vi "test_output_freq_fpga.vi"() -> ()   [LabVIEW 2013]
uses:
  <vilib>/Platform/TimedLoop/XDataNode/timing_clust.ctl
  <vilib>/Platform/TimedLoop/XDataNode/nitl_modes.ctl
  <vilib>/Platform/TimedLoop/XDataNode/wakeup.ctl
  <vilib>/rvi/Emulation/niFpgaSctlEmulationGetInTimedLoop.vi
  <vilib>/rvi/Emulation/niFpgaEmulationReportErrorSimple.vi
  <vilib>/rvi/Emulation/niFpgaGetClockAttributes.vi
  <vilib>/rvi/eio/common/nirviEmuTemplateMethod_errors.vi
  <vilib>/rvi/Emulation/niFpgaCriticalErrorInLSC.vi
  <vilib>/Platform/TimedLoop/XDataNode/XDataNode.xnode
  <vilib>/eio/EIONode/EIONode.xnode
  <vilib>/rvi/FXPMathLib/FxpSub/XNode/nifxpmath_Sub.xnode
  <vilib>/Platform/TimedLoop/XDataNode/XDNodeRunTimeDep.lvlib
  <vilib>/rvi/FXPMathLib/sim/FxpSim.dll
panel:
  in  "samples per period":fxp<+,32,32>=1000000000.0
  in  "set samples":bool
  in  "User Command Commit":bool
  in  "User Command":u8
  out "User Command Idle":bool
  out "User Command Status":u8
  in  "User Data 0":u8
  in  "User Data 1":u8
  out "PLL Locked":bool
  out "User Error":bool
  out "Configured?":bool
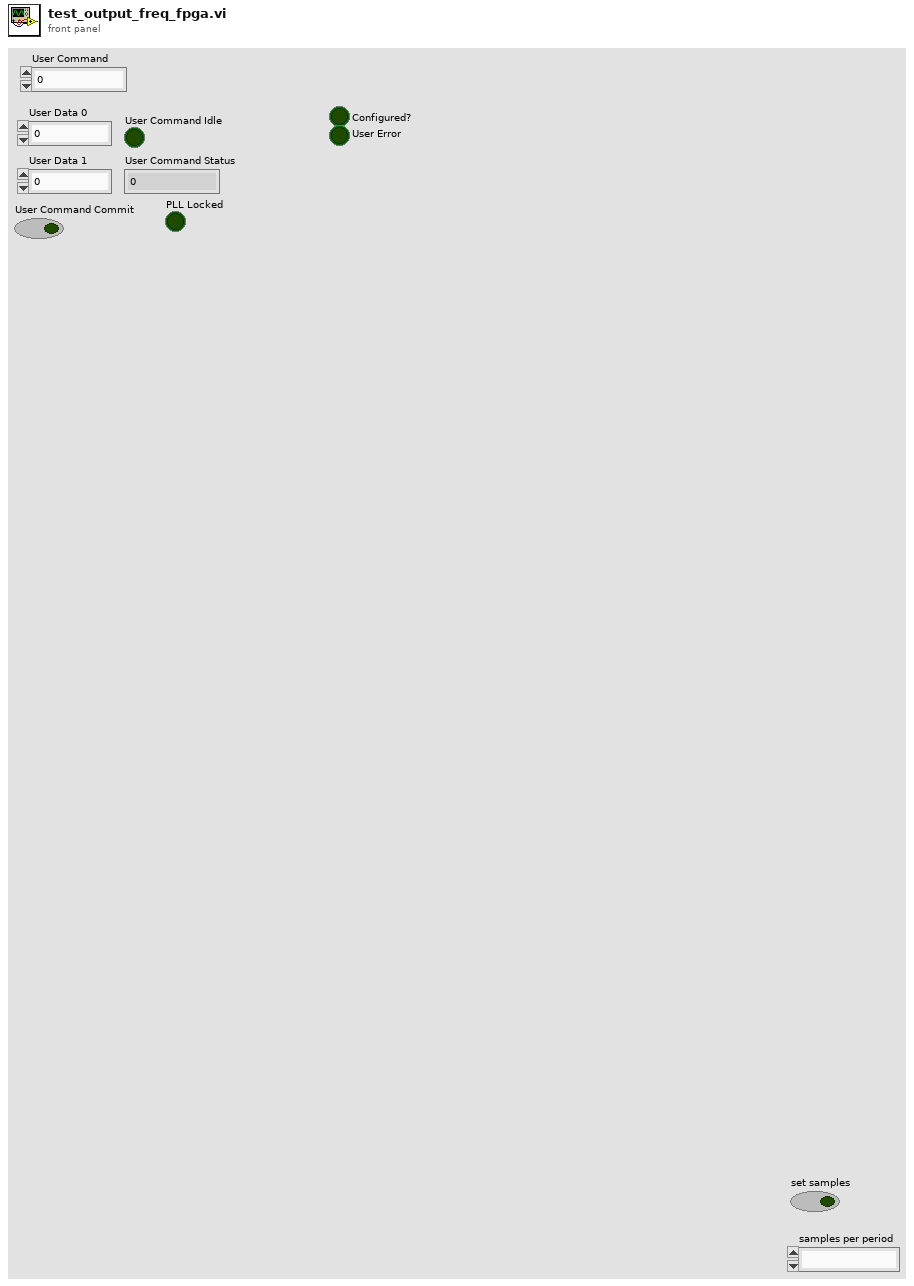
[diagram p1: front panel]
types:
  T1 = typedef "XDNodeRunTimeDep.lvlib/timing_clust.ctl" = cluster{"Expected End [f-1]":u64, "Actual End [f-1]":u64, "Finished Late? [f-1]":bool, "Expected End [i-1]":u64, "Actual End [i-1]":u64, "Finished Late? [i-1]":bool, "Expected Start [i]":u64, "Actual Start [i]":u64, "Expected Start [f]":u64, "Actual Start [f]":u64, "Source Name":string, "Structure Name":string, "Period":i64, "Deadline":i64, "Offset":i64, "Start":i64, "Priority":i32, "Timeout":i32, "Mode":T2, "Wakeup Reason":T3, "Error":errorcluster, "Source Type":string, "Secondary Source Type":string, "Global End Time":u64, "Global Start Time":u64, "Frame Duration":u64, "Iteration Duration":u64, "Assigned CPU":i32, "I/O Scan Engine Mode":u32}
  T2 = typedef "XDNodeRunTimeDep.lvlib/nitl_modes.ctl" = enum32{"No Change", "Process missed periods, maintain original phase", "Discard missed periods, maintain original phase", "Process missed periods, ignore original phase", "Discard missed periods, ignore original phase"}
  T3 = typedef "XDNodeRunTimeDep.lvlib/wakeup.ctl" = enum32{"Normal", "Aborted", "Asynchronous wakeup", "Timing source error", "Timed loop error", "Timeout"}
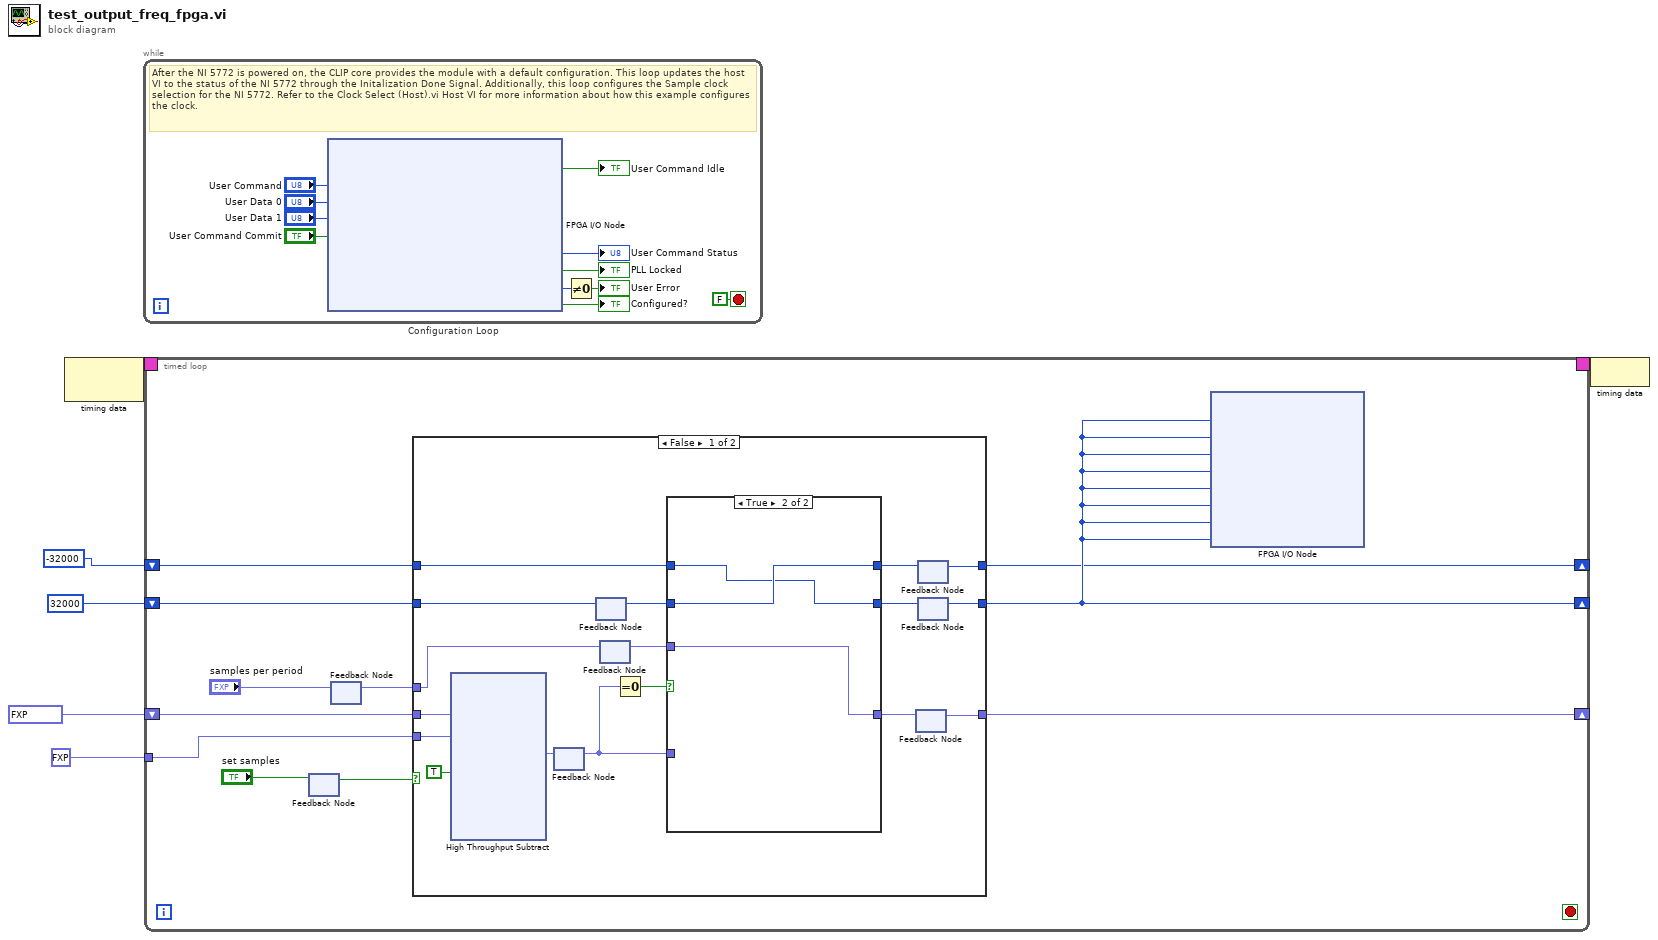
[diagram p0: block diagram]
diagram:
  n1 = node-c288() -> (w6:T1)  [unwired: 1 in]
  n2 = while "Configuration Loop" {
    stop <- FALSE stop-if-true
    # "After the NI 5772 is powered on, the CLIP core provides the module with a default configuration. This loop updates the host VI to the status of the NI 5772 through the Initalization Done Signal. Additionally, this loop configures the Sample clock selection for the NI 5772. Refer to the Clock Select (Host).vi Host VI for more information about how this example configures the clock."
    n3 = xnode "FPGA I/O Node"("IO Module\\User Command"="User Command", "IO Module\\User Data 0"="User Data 0", "IO Module\\User Data 1"="User Data 1", "IO Module\\User Command Commit"="User Command Commit") -> ("IO Module\\User Command Idle"=→"User Command Idle":bool, "IO Module\\User Command Status"=→"User Command Status":u8, "IO Module\\PLL Locked"=→"PLL Locked":bool, "IO Module\\User Error"=w12:u8, "IO Module\\Initialization Done"=→"Configured?":bool)  [unwired: 9 in, 9 out]
    n4 = Not Equal To 0?(x=w12) -> (x != 0?=→"User Error":bool)
  }
  n5 = timed-loop {
    timing: w6 -> [_]
    timing-out: [_] -> w5
    shift-right: [w24] -> _
    shift-left: i16 32000 ("samples per period") -> [w26]
    shift-right: [w25] -> _
    shift-left: fxp<+,32,32> 50000000.0 ("samples per period") -> [w28]
    tunnel: fxp<+,32,32> 1.0 ("samples per period") -> [w27]
    shift-right: [w18] -> _
    shift-left: i16 -32000 ("samples per period") -> [w19]
    stop <- _ stop-if-true
    n6 = feedback #1() -> (w22:bool)  [unwired: 1 in]
    n7 = feedback-in #1("set samples") -> ()
    n8 = feedback #2() -> (w20:fxp<+,32,32>)  [unwired: 1 in]
    n9 = feedback-in #2("samples per period") -> ()
    n10 = case shown="False" w22 {
      tunnel: w28 -> [w44 _]
      tunnel: w20 -> [w36 w54]
      tunnel: w27 -> [w45 _]
      tunnel: w26 -> [w38 w53]
      tunnel: [w39 w54] -> w25
      tunnel: [w41 w53] -> w24
      tunnel: w19 -> [w31 w52]
      tunnel: [w29 w52] -> w18
      frame False {
        n11 = xnode "High Throughput Subtract"("x"=w44, "y"=w45, "input valid"=TRUE) -> ("x-y"=w34:fxp<+,32,32>)  [unwired: 1 in, 2 out]
        n12 = feedback #3() -> (w33:fxp<+,32,32>)  [unwired: 1 in]
        n13 = feedback-in #3(w34) -> ()
        n14 = feedback #4() -> (w37:i16)  [unwired: 1 in]
        n15 = feedback-in #4(w38) -> ()
        n16 = feedback #5() -> (w35:fxp<+,32,32>)  [unwired: 1 in]
        n17 = feedback-in #5(w36) -> ()
        n18 = Equal To 0?(x=w33) -> (x = 0?=w43:bool)
        n19 = case shown="True" w43 {
          tunnel: w35 -> [_ w51]
          tunnel: [w48 w51] -> w40
          tunnel: w33 -> [w48 _]
          tunnel: w37 -> [w46 w50]
          tunnel: [w46 w49] -> w42
          tunnel: [w47 w50] -> w30
          tunnel: w31 -> [w47 w49]
          frame False {
          }
          frame True {
          }
        }
        n20 = feedback #6() -> (w39:fxp<+,32,32>)  [unwired: 1 in]
        n21 = feedback-in #6(w40) -> ()
        n22 = feedback #7() -> (w29:i16)  [unwired: 1 in]
        n23 = feedback-in #7(w30) -> ()
        n24 = feedback #8() -> (w41:i16)  [unwired: 1 in]
        n25 = feedback-in #8(w42) -> ()
      }
      frame True {
      }
    }
    n26 = xnode "FPGA I/O Node"("IO Module\\AO 0 N-3"=w24, "IO Module\\AO 0 N-2"=w24, "IO Module\\AO 0 N-1"=w24, "IO Module\\AO 0 N"=w24, "IO Module\\AO 1 N-3"=w24, "IO Module\\AO 1 N-2"=w24, "IO Module\\AO 1 N-1"=w24, "IO Module\\AO 1 N"=w24) -> ()  [unwired: 8 in, 8 out]
  }
  n27 = node-c288(w5) -> ()
